vi "VFDSampleSensorLoop.vi"   [LabVIEW 2018]
uses:
  VFDSampleSensorLoopData.ctl
  VFDSampleSensorLoopStates.ctl
  VFDSample.ctl
  VFDErrorSample.ctl
  VFDErrorCodes.ctl
  <vilib>/Platform/TimedLoop/XDataNode/timing_clust.ctl
  <vilib>/Platform/TimedLoop/XDataNode/nitl_modes.ctl
  <vilib>/Platform/TimedLoop/XDataNode/wakeup.ctl
  <vilib>/rvi/Emulation/niFpgaSctlEmulationGetInTimedLoop.vi
  <vilib>/rvi/Emulation/niFpgaEmulationReportErrorSimple.vi
  <vilib>/rvi/Emulation/niFpgaGetClockAttributes.vi
  <vilib>/rvi/Emulation/niFpgaCriticalErrorInLSC.vi
  <vilib>/rvi/Emulation/niFpgaEmulationIsFPGAContextNoSignature.vi
  <vilib>/rvi/errors/niFpgaSetErrorForExecOnDevCompSimple.vi
  <vilib>/rvi/eio/common/nirviEmuReportErrorAndStop.vi
  <vilib>/rvi/DataTransferAndStorage/Container/Common/niFpgaContainerGetUniqueNameForEmu.vi
  <vilib>/rvi/FIFO/Fifo_Resource/nirvififoEmulationSetSize.vi
  <vilib>/rvi/FIFO/Fifo_Resource/nirviFifoEmulationQueueMgr.vi
  <instcachedir>/0/nirviFifoEmulationQueueMgr_E5CAEC123FF24DC58D834DCA3CDAA9B5.lvgen/nirviFifoEmulationQueueMgr_E5CAEC123FF24DC58D834DCA3CDAA9B5_002.vi
  <vilib>/Utility/error.llb/Clear Errors.vi
  <vilib>/rvi/FIFO/Fifo_Resource/nirvififoEmulationCreateLock.vi
  <vilib>/rvi/Emulation/niFpgaProcessEmulError.vi
  <vilib>/rvi/FIFO/Fifo_Resource/nirvififoEmulationObtainLock.vi
  <vilib>/rvi/FIFO/Fifo_Resource/nirvififoEmulationReleaseLock.vi
  <vilib>/rvi/occurrence/nirviWaitOnOccurrenceBase.vi
  <vilib>/rvi/errors/nirviReportUnexpectedCaseInternalError.vi
  <vilib>/rvi/errors/nirviReportUnexpectedCaseInternalError (U32).vi
  <vilib>/rvi/FIFO/Fifo_Resource/nirvififoEmulationDetermineInputValidOut.vi
  <instcachedir>/0/nirviFifoEmulationQueueMgr_E5CAEC123FF24DC58D834DCA3CDAA9B5.lvgen/nirviFifoEmulationQueueMgr_E5CAEC123FF24DC58D834DCA3CDAA9B5_001.vi
  <instcachedir>/0/nirviFifoEmulationQueueMgr_E5CAEC123FF24DC58D834DCA3CDAA9B5.lvgen/nirviFifoEmulationQueueMgr_E5CAEC123FF24DC58D834DCA3CDAA9B5_004.vi
  <vilib>/rvi/Memory/Memory_Emulation/niFpgaMemoryEmulationCacheClearOnFirstRun.vi
  <vilib>/rvi/Memory/Memory_Emulation/nirvimemoryEmulationManagerCache_MakeExclusive.vi
  <vilib>/rvi/Memory/Memory_Emulation/niFpgaMemoryEmulationValidateCache.vi
  <vilib>/rvi/Memory/Memory_Emulation/nirvimemoryEmulationManagerCache_InsertValue.vi
  <vilib>/rvi/Memory/Memory_Emulation/nirvimemoryEmulationManagerCache_ReleaseExclusive.vi
  <vilib>/rvi/Memory/Memory_Emulation/nirvimemoryEmulationManagerCache_GetValue.vi
  <vilib>/rvi/Memory/Memory_Emulation/nirvimemoryEmulationManagerCache_SetValue.vi
  <instcachedir>/0/nirviFifoEmulationQueueMgr_E5CAEC123FF24DC58D834DCA3CDAA9B5.lvgen/nirviFifoEmulationQueueMgr_E5CAEC123FF24DC58D834DCA3CDAA9B5_029.vi
  <instcachedir>/0/nirviFifoEmulationQueueMgr_E5CAEC123FF24DC58D834DCA3CDAA9B5.lvgen/nirviFifoEmulationQueueMgr_E5CAEC123FF24DC58D834DCA3CDAA9B5_015.vi
  <vilib>/Platform/TimedLoop/XDataNode/XDataNode.xnode
  <vilib>/rvi/DataTransferAndStorage/Container/XNode/niFpgaContainer.xnode
  <vilib>/rvi/FIFO/Fifo_Resource/nirvififoEmulationRead.vi
  <vilib>/rvi/FIFO/Fifo_Resource/nirvififoEmulationWrite.vi
  <vilib>/rvi/DataTransferAndStorage/Register/Emulation/niFpgaRegisterEmulation.vi
  <vilib>/Platform/TimedLoop/XDataNode/XDNodeRunTimeDep.lvlib
types:
  T1 = typedef "VFDSampleSensorLoopData.ctl" = cluster{"State":T2, "StateAfterRead":T2, "Timestamp":u64, "Timeout":i32, "U16":u16, "CRC":u16, "Exception":u8, "Sample":T3, "ErrorSample":T4}
  T2 = typedef "VFDSampleSensorLoopStates.ctl" = enum16{"WaitForTrigger", "ClearRxFIFO", "WaitForClearComplete", "WriteAddress", "WriteFunction", "WriteStartAddress1", "WriteStartAddress0", "WriteAddressCount1", "WriteAddressCount0", "WriteCRC1", "WriteCRC0", "ReadAddress", "ReadFunction", "ReadByteCount", "StartVelocityBits", "EndVelocityBits", "StartDriveErrorBits", "EndDriveErrorBits", "StartFrequencyCommand", "EndFrequencyCommand", "StartOutputFrequency", "EndOutputFrequency", "StartOutputCurrent", "EndOutputCurrent", "StartDCBusVoltage", "EndDCBusVoltage", "StartOutputVoltage", "EndOutputVoltage", "ReadDataByte1", "ReadDataByte0", "Reserved1", "Reserved2", "ReadCRCByte0", "ReadCRCByte1", "CalculateCRC", "ValidateCRC", "PrepareSample", "MoveSample", "ReadExceptionCode", "ReadExceptionCRCByte0", "ReadExceptionCRCByte1", "CalculateExceptionCRC", "ValidateExceptionCRC", "ParseExceptionCode", "ResponseAddressError", "ResponseFunctionCodeError", "ResponseByteCountError", "ResponseCRCError", "ResponseUnknownError", "ResponseTimeoutError", "SensorReportsIllegalFunction", "SensorReportsIllegalDataAddress", "PrepareErrorCode", "MoveErrorCode", "WriteDemandAddress", "WriteDemandFunction", "WriteDemandStartAddress1", "WriteDemandStartAddress0", "WriteDemandData1", "WriteDemandData0", "CalculateDemandCRC", "WaitForDemandCRC", "WriteDemandCRC1", "WriteDemandCRC0", "ReadDemandAddress", "ReadDemandFunction", "ReadDemandStartAddress1", "ReadDemandStartAddress0", "ReadDemandData1", "ReadDemandData0", "ReadDemandCRC0", "ReadDemandCRC1", "CalculateDemandResponseCRC", "ValidateDemandResponseCRC"}
  T3 = typedef "VFDSample.ctl" = cluster{"Timestamp":u64, "TxBytes":u64, "RxBytes":u64, "TxFrames":u64, "RxFrames":u64, "VelocityBits":u16, "DriveErrorBits":u16, "FrequencyCommand":u16, "OutputFrequency":u16, "OutputCurrent":u16, "DCBusVoltage":u16, "OutputVoltage":u16}
  T4 = typedef "VFDErrorSample.ctl" = cluster{"Timestamp":u64, "TxBytes":u64, "RxBytes":u64, "TxFrames":u64, "RxFrames":u64, "ErrorCode":T5}
  T5 = typedef "VFDErrorCodes.ctl" = enum8{"None", "ResponseAddressError", "ResponseFunctionCodeError", "ResponseByteCountError", "ResponseCRCError", "ResponseUnknownError", "ResponseTimeoutError", "SensorReportsIllegalFunction", "SensorReportsIllegalDataAddress"}
  T6 = typedef "XDNodeRunTimeDep.lvlib/timing_clust.ctl" = cluster{"Expected End [f-1]":u64, "Actual End [f-1]":u64, "Finished Late? [f-1]":bool, "Expected End [i-1]":u64, "Actual End [i-1]":u64, "Finished Late? [i-1]":bool, "Expected Start [i]":u64, "Actual Start [i]":u64, "Expected Start [f]":u64, "Actual Start [f]":u64, "Source Name":string, "Structure Name":string, "Period":i64, "Deadline":i64, "Offset":i64, "Start":i64, "Priority":i32, "Timeout":i32, "Mode":T7, "Wakeup Reason":T8, "Error":errorcluster, "Source Type":string, "Secondary Source Type":string, "Global End Time":u64, "Global Start Time":u64, "Frame Duration":u64, "Iteration Duration":u64, "Assigned CPU":i32, "I/O Scan Engine Mode":u32}
  T7 = typedef "XDNodeRunTimeDep.lvlib/nitl_modes.ctl" = enum32{"No Change", "Process missed periods, maintain original phase", "Discard missed periods, maintain original phase", "Process missed periods, ignore original phase", "Discard missed periods, ignore original phase"}
  T8 = typedef "XDNodeRunTimeDep.lvlib/wakeup.ctl" = enum32{"Normal", "Aborted", "Asynchronous wakeup", "Timing source error", "Timed loop error", "Timeout"}
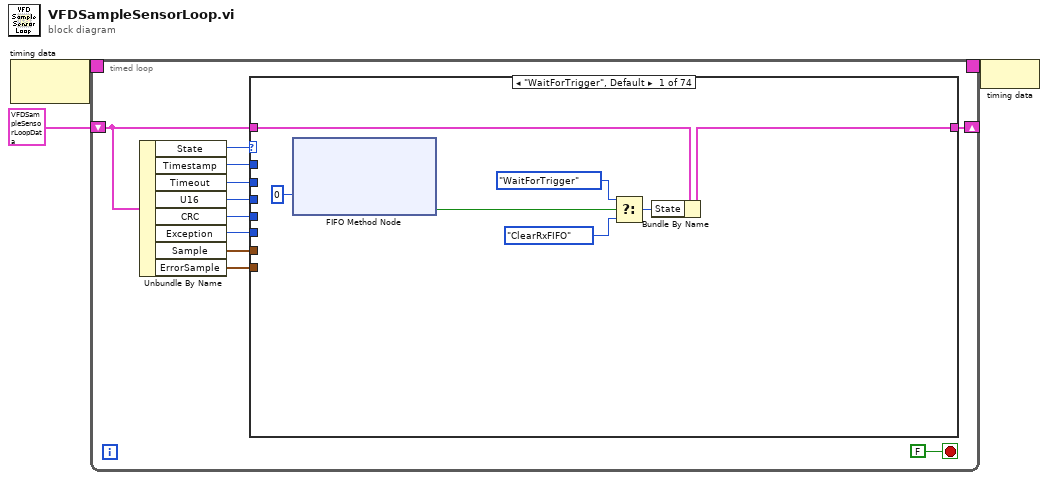
[diagram p0: block diagram]
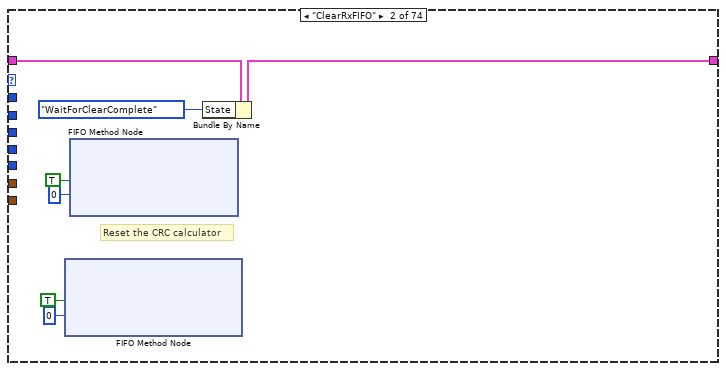
[diagram p2: hidden frame]
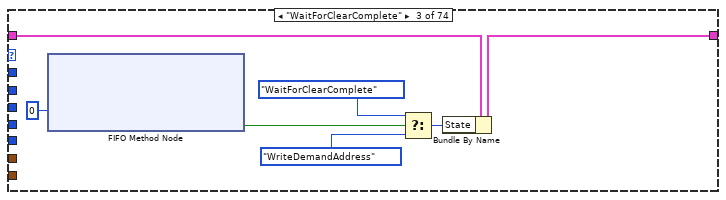
[diagram p3: hidden frame]
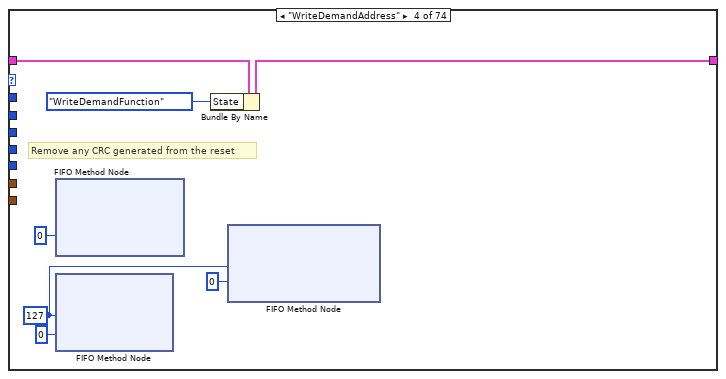
[diagram p4: hidden frame]
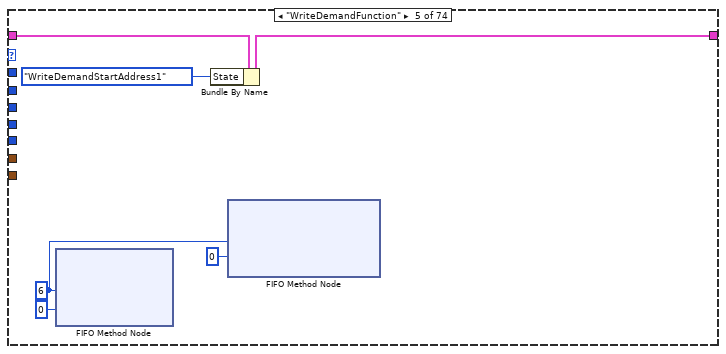
[diagram p5: hidden frame]
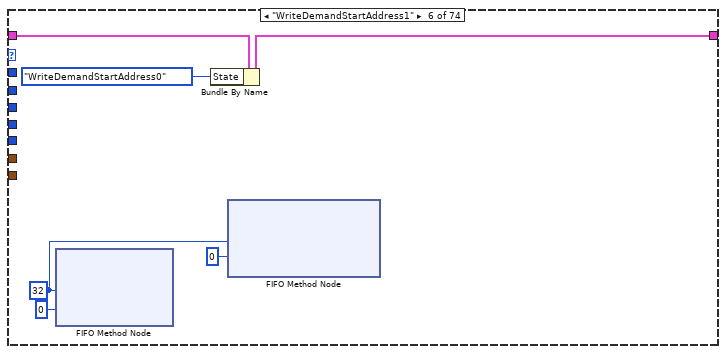
[diagram p6: hidden frame]
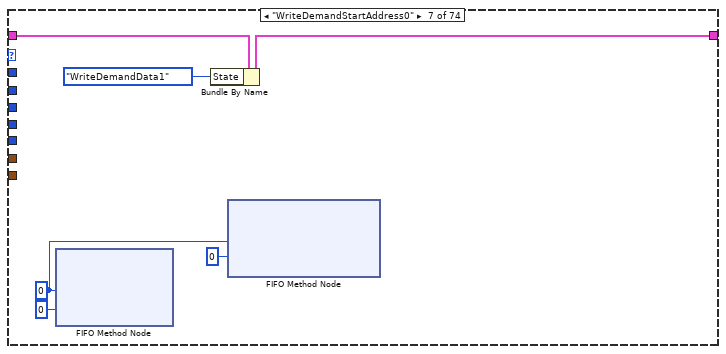
[diagram p7: hidden frame]
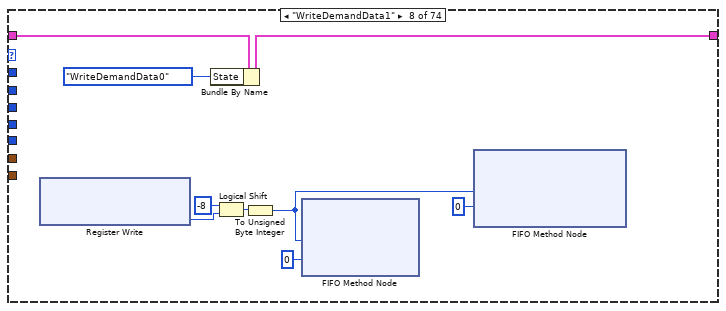
[diagram p8: hidden frame]
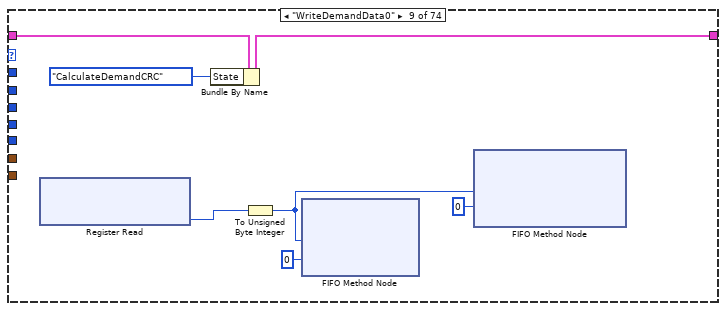
[diagram p9: hidden frame]
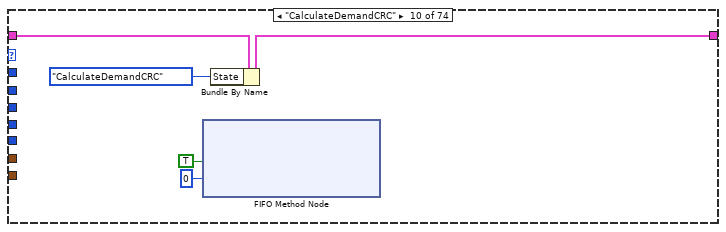
[diagram p10: hidden frame]
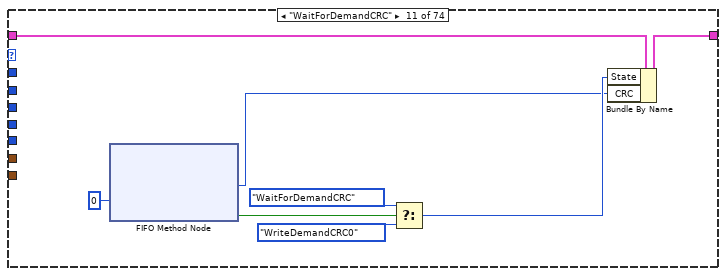
[diagram p11: hidden frame]
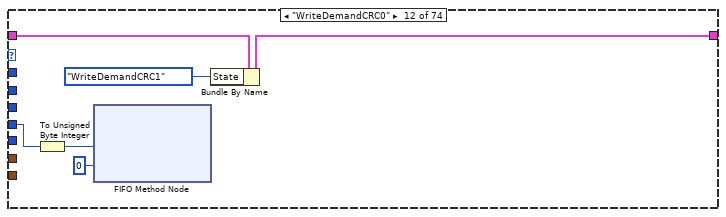
[diagram p12: hidden frame]
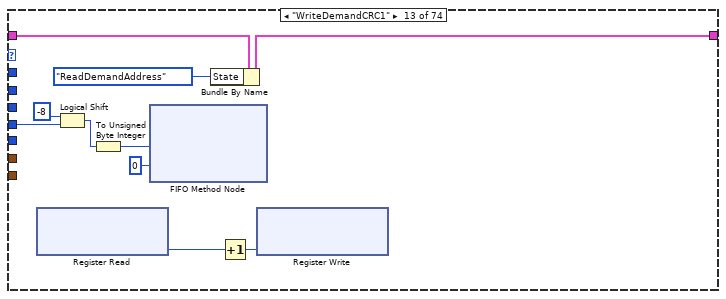
[diagram p13: hidden frame]
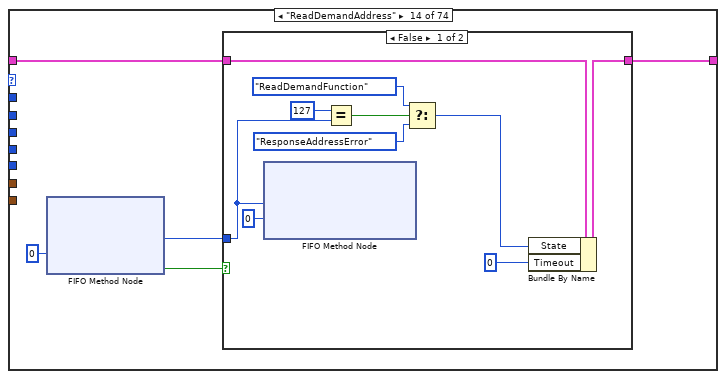
[diagram p14: hidden frame]
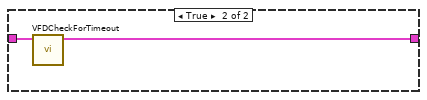
[diagram p15: hidden frame]
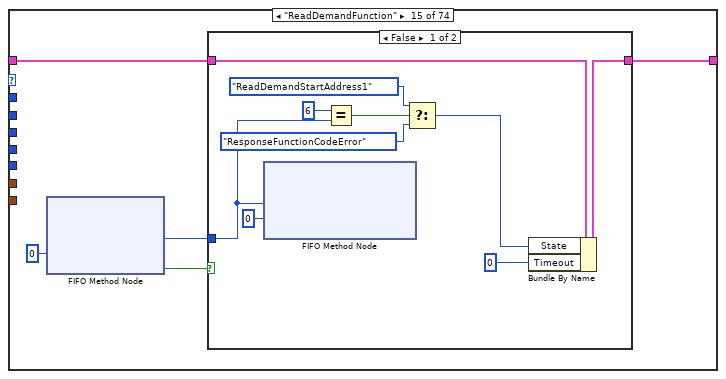
[diagram p16: hidden frame]
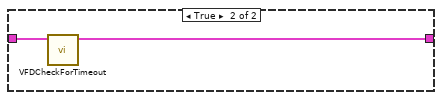
[diagram p17: hidden frame]
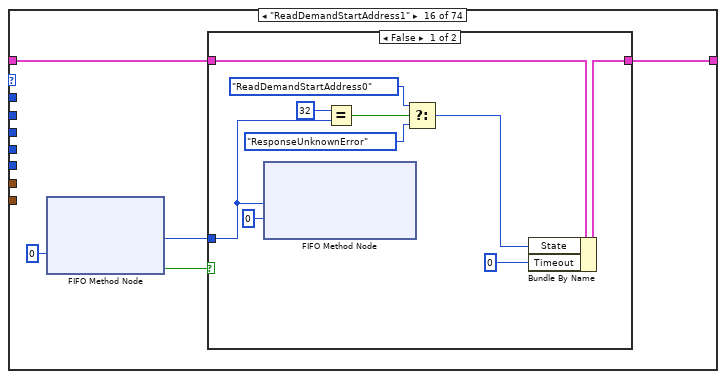
[diagram p18: hidden frame]
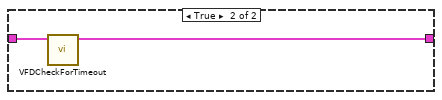
[diagram p19: hidden frame]
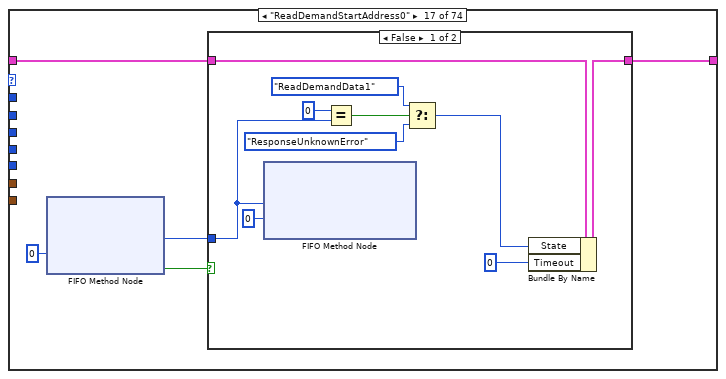
[diagram p20: hidden frame]
diagram:
  n1 = node-c288() -> (w3:T6)  [unwired: 1 in]
  n2 = timed-loop {
    timing: w3 -> [_]
    timing-out: [_] -> w2
    shift-right: [w13] -> _
    shift-left: T1 {"State"=enum."WaitForTrigger", "StateAfterRead"=enum."ClearRxFIFO", "Timestamp"=0, "Timeout"=0, "U16"=0, "CRC"=0, "Exception"=0, "Sample"={"Timestamp"=0, "TxBytes"=0, "RxBytes"=0, "TxFrames"=0, "RxFrames"=0, "VelocityBits"=0, "DriveErrorBits"=0, "FrequencyCommand"=0, "OutputFrequency"=0, "OutputCurrent"=0, "DCBusVoltage"=0, "OutputVoltage"=0}, "ErrorSample"={"Timestamp"=0, "TxBytes"=0, "RxBytes"=0, "TxFrames"=0, "RxFrames"=0, "ErrorCode"=enum."None"}} ("InclinometerData") -> [w14]
    stop <- FALSE stop-if-true
    n3 = Unbundle By Name(w14) -> ("State"=w12:T2, "Timestamp"=w7:u64, "Timeout"=w11:i32, "U16"=w10:u16, "CRC"=w9:u16, "Exception"=w6:u8, "Sample"=w5:T3, "ErrorSample"=w4:T4)
    n4 = case shown="\"WaitForTrigger\", Default" w12 {
      tunnel: w14 -> [w20 w27 w34 w41 w47 w53 w59 w68 w75 w80 w88 w94 w104 w106 w123 w140 w157 w174 w194 w212 w227 w247 w250 w271 w276 w281 w286 w291 w296 w301 w309 w313 w330 w351 w372 w376 w381 w385 w390 w394 w399 w403 w408 w412 w417 w421 w426 w430 w432 w455 w474 w477 w482 w502 w522 w527 w547 w552 w556 w577 w597 w617 w622 w642 w646 w650 w654 w658 w662 w666 w670 w674 w682 w687]
      tunnel: [w21 w28 w35 w42 w48 w54 w60 w69 w76 w81 w89 w95 w105 w107 w124 w141 w158 w175 w195 w213 w228 w245 w251 w272 w277 w282 w287 w292 w297 w302 w310 w314 w331 w352 w371 w375 w380 w384 w389 w393 w398 w402 w407 w411 w416 w420 w425 w429 w433 w456 w475 w478 w483 w503 w523 w528 w548 w553 w557 w578 w598 w618 w623 w643 w647 w651 w655 w659 w663 w667 w671 w675 w683 w688] -> w13
      tunnel: w11 -> [_ _ _ _ _ _ _ _ _ _ _ _ _ _ _ _ _ _ _ _ _ _ _ _ _ _ _ _ _ _ _ _ _ _ _ _ _ _ _ _ _ _ _ _ _ _ _ _ _ _ _ _ _ _ _ _ _ _ _ _ _ _ _ _ _ _ _ _ _ _ _ _ _ _]
      tunnel: w10 -> [_ _ _ _ _ _ _ _ _ _ _ _ _ _ _ _ _ _ _ _ _ _ _ _ _ _ _ _ _ _ _ _ _ _ _ w373 _ w382 _ w391 _ w400 _ w409 _ w418 _ w427 w431 w454 _ _ _ _ _ _ _ _ _ _ _ _ _ _ _ _ _ _ _ _ _ _ _ _]
      tunnel: w9 -> [_ _ _ _ _ _ _ _ _ _ _ w90 w100 _ _ _ _ _ _ _ w226 _ w249 _ _ _ _ _ _ _ _ _ _ _ _ _ _ _ _ _ _ _ _ _ _ _ _ _ _ _ _ _ w481 w501 _ w526 _ _ _ w576 w596 _ w621 _ _ _ _ _ _ _ _ _ _ _]
      tunnel: w7 -> [_ _ _ _ _ _ _ _ _ _ _ _ _ _ _ _ _ _ _ _ _ _ _ _ _ _ _ _ _ _ _ _ _ _ _ _ _ _ _ _ _ _ _ _ _ _ _ _ _ _ _ _ _ _ _ _ w546 _ _ _ _ _ _ _ _ _ _ _ _ _ _ _ w681 _]
      tunnel: w6 -> [_ _ _ _ _ _ _ _ _ _ _ _ _ _ _ _ _ _ _ _ _ _ _ _ _ _ _ _ _ _ _ _ _ _ _ _ _ _ _ _ _ _ _ _ _ _ _ _ _ _ _ _ _ _ _ _ _ _ _ _ _ _ _ w637 _ _ _ _ _ _ _ _ _ _]
      tunnel: w5 -> [_ _ _ _ _ _ _ _ _ _ _ _ _ _ _ _ _ _ _ _ _ _ _ _ _ _ _ _ _ _ _ _ _ _ _ _ _ _ _ _ _ _ _ _ _ _ _ _ _ _ _ _ _ _ _ _ _ w549 _ _ _ _ _ _ _ _ _ _ _ _ _ _ _ _]
      tunnel: w4 -> [_ _ _ _ _ _ _ _ _ _ _ _ _ _ _ _ _ _ _ _ _ _ _ _ _ _ _ _ _ _ _ _ _ _ _ _ _ _ _ _ _ _ _ _ _ _ _ _ _ _ _ _ _ _ _ _ _ _ _ _ _ _ _ _ _ _ _ _ _ _ _ _ _ w685]
      frame "WaitForTrigger", Default {
        n5 = xnode ("FIFO Method Node")("Timeout"=0) -> ("Timed Out?"=w15:bool)  [unwired: 1 in, 2 out]
        n6 = Select(t=VFDSampleSensorLoopStates."WaitForTrigger" ("InclinometerState"), s=w15, f=VFDSampleSensorLoopStates."ClearRxFIFO" ("InclinometerState")) -> (s? t:f=w17:T2)
        n7 = Bundle By Name(cluster=w20, "State"=w17) -> (w21:T1)
      }
      frame "ClearRxFIFO" {
        # "Reset the CRC calculator"
        n8 = xnode ("FIFO Method Node")("Element"=TRUE, "Timeout"=0) -> ()  [unwired: 1 in, 2 out]
        n9 = xnode ("FIFO Method Node")("Element"=TRUE, "Timeout"=0) -> ()  [unwired: 1 in, 2 out]
        n10 = Bundle By Name(cluster=w27, "State"=VFDSampleSensorLoopStates."WaitForClearComplete" ("InclinometerState")) -> (w28:T1)
      }
      frame "WaitForClearComplete" {
        n11 = xnode ("FIFO Method Node")("Timeout"=0) -> ("Timed Out?"=w29:bool)  [unwired: 1 in, 2 out]
        n12 = Select(t=VFDSampleSensorLoopStates."WaitForClearComplete", s=w29, f=VFDSampleSensorLoopStates."WriteDemandAddress" ("InclinometerState")) -> (s? t:f=w31:T2)
        n13 = Bundle By Name(cluster=w34, "State"=w31) -> (w35:T1)
      }
      frame "WriteDemandAddress" {
        w37 = u8 127 ("Element")
        # "Remove any CRC generated from the reset"
        n14 = xnode ("FIFO Method Node")("Timeout"=0) -> ()  [unwired: 1 in, 3 out]
        n15 = xnode ("FIFO Method Node")("Element"=w37, "Timeout"=0) -> ()  [unwired: 1 in, 2 out]
        n16 = Bundle By Name(cluster=w41, "State"=VFDSampleSensorLoopStates."WriteDemandFunction" ("InclinometerState")) -> (w42:T1)
        n17 = xnode ("FIFO Method Node")("Element"=w37, "Timeout"=0) -> ()  [unwired: 1 in, 2 out]
      }
      frame "WriteDemandFunction" {
        w44 = u8 6 ("Element")
        n18 = xnode ("FIFO Method Node")("Element"=w44, "Timeout"=0) -> ()  [unwired: 1 in, 2 out]
        n19 = Bundle By Name(cluster=w47, "State"=VFDSampleSensorLoopStates."WriteDemandStartAddress1" ("InclinometerState")) -> (w48:T1)
        n20 = xnode ("FIFO Method Node")("Element"=w44, "Timeout"=0) -> ()  [unwired: 1 in, 2 out]
      }
      frame "WriteDemandStartAddress1" {
        w50 = u8 32 ("Element")
        n21 = xnode ("FIFO Method Node")("Element"=w50, "Timeout"=0) -> ()  [unwired: 1 in, 2 out]
        n22 = Bundle By Name(cluster=w53, "State"=VFDSampleSensorLoopStates."WriteDemandStartAddress0" ("InclinometerState")) -> (w54:T1)
        n23 = xnode ("FIFO Method Node")("Element"=w50, "Timeout"=0) -> ()  [unwired: 1 in, 2 out]
      }
      frame "WriteDemandStartAddress0" {
        w56 = u8 0 ("Element")
        n24 = xnode ("FIFO Method Node")("Element"=w56, "Timeout"=0) -> ()  [unwired: 1 in, 2 out]
        n25 = Bundle By Name(cluster=w59, "State"=VFDSampleSensorLoopStates."WriteDemandData1" ("InclinometerState")) -> (w60:T1)
        n26 = xnode ("FIFO Method Node")("Element"=w56, "Timeout"=0) -> ()  [unwired: 1 in, 2 out]
      }
      frame "WriteDemandData1" {
        n27 = xnode "Register Write"() -> ("Data"=w64:u16)  [unwired: 1 in, 1 out]
        n28 = Bundle By Name(cluster=w68, "State"=VFDSampleSensorLoopStates."WriteDemandData0" ("InclinometerState")) -> (w69:T1)
        n29 = Logical Shift(y=i16 -8, x=w64) -> (x << y=w62:u16)
        n30 = To Unsigned Byte Integer(number=w62) -> (unsigned 8bit integer=w61:u8)
        n31 = xnode ("FIFO Method Node")("Element"=w61, "Timeout"=0) -> ()  [unwired: 1 in, 2 out]
        n32 = xnode ("FIFO Method Node")("Element"=w61, "Timeout"=0) -> ()  [unwired: 1 in, 2 out]
      }
      frame "WriteDemandData0" {
        n33 = xnode "Register Read"() -> ("Data"=w70:u16)  [unwired: 1 in, 1 out]
        n34 = Bundle By Name(cluster=w75, "State"=VFDSampleSensorLoopStates."CalculateDemandCRC" ("InclinometerState")) -> (w76:T1)
        n35 = To Unsigned Byte Integer(number=w70) -> (unsigned 8bit integer=w71:u8)
        n36 = xnode ("FIFO Method Node")("Element"=w71, "Timeout"=0) -> ()  [unwired: 1 in, 2 out]
        n37 = xnode ("FIFO Method Node")("Element"=w71, "Timeout"=0) -> ()  [unwired: 1 in, 2 out]
      }
      frame "CalculateDemandCRC" {
        n38 = xnode ("FIFO Method Node")("Element"=TRUE, "Timeout"=0) -> ()  [unwired: 1 in, 2 out]
        n39 = Bundle By Name(cluster=w80, "State"=VFDSampleSensorLoopStates."CalculateDemandCRC" ("InclinometerState")) -> (w81:T1)
      }
      frame "WaitForDemandCRC" {
        n40 = xnode ("FIFO Method Node")("Timeout"=0) -> ("Element"=w82:u16, "Timed Out?"=w87:bool)  [unwired: 1 in, 1 out]
        n41 = Select(t=VFDSampleSensorLoopStates."WaitForDemandCRC", s=w87, f=VFDSampleSensorLoopStates."WriteDemandCRC0" ("InclinometerState")) -> (s? t:f=w83:T2)
        n42 = Bundle By Name(cluster=w88, "State"=w83, "CRC"=w82) -> (w89:T1)
      }
      frame "WriteDemandCRC0" {
        n43 = To Unsigned Byte Integer(number=w90) -> (unsigned 8bit integer=w91:u8)
        n44 = xnode ("FIFO Method Node")("Element"=w91, "Timeout"=0) -> ()  [unwired: 1 in, 2 out]
        n45 = Bundle By Name(cluster=w94, "State"=VFDSampleSensorLoopStates."WriteDemandCRC1" ("InclinometerState")) -> (w95:T1)
      }
      frame "WriteDemandCRC1" {
        n46 = xnode ("Register Read")() -> ("Data"=w97:u64)  [unwired: 1 in, 1 out]
        n47 = Logical Shift(y=i16 -8, x=w100) -> (x << y=w98:u16)
        n48 = To Unsigned Byte Integer(number=w98) -> (unsigned 8bit integer=w101:u8)
        n49 = xnode ("FIFO Method Node")("Element"=w101, "Timeout"=0) -> ()  [unwired: 1 in, 2 out]
        n50 = Bundle By Name(cluster=w104, "State"=VFDSampleSensorLoopStates."ReadDemandAddress" ("InclinometerState")) -> (w105:T1)
        n51 = Increment(x=w97) -> (x+1=w96:u64)
        n52 = xnode ("Register Write")("Data"=w96) -> ()  [unwired: 1 in, 1 out]
      }
      frame "ReadDemandAddress" {
        n53 = xnode ("FIFO Method Node")("Timeout"=0) -> ("Element"=w108:u8, "Timed Out?"=w109:bool)  [unwired: 1 in, 1 out]
        n54 = case shown="False" w109 {
          tunnel: w108 -> [w117 _]
          tunnel: [w119 w121] -> w107
          tunnel: w106 -> [w120 w122]
          frame False {
            n55 = xnode ("FIFO Method Node")("Element"=w117, "Timeout"=0) -> ()  [unwired: 1 in, 2 out]
            n56 = Equal?(x=u8 127, y=w117) -> (x = y?=w115:bool)
            n57 = Select(t=VFDSampleSensorLoopStates."ReadDemandFunction" ("InclinometerState"), s=w115, f=VFDSampleSensorLoopStates."ResponseAddressError" ("InclinometerState")) -> (s? t:f=w112:T2)
            n58 = Bundle By Name(cluster=w120, "State"=w112, "Timeout"=0) -> (w119:T1)
          }
          frame True {
            n59 = call "VFDCheckForTimeout.vi"("VFDSampleSensorLoopData in"=w122) -> ("VFDSampleSensorLoopData out"=w121:T1)  [unwired: 10 in]
          }
        }
      }
      frame "ReadDemandFunction" {
        n60 = xnode ("FIFO Method Node")("Timeout"=0) -> ("Element"=w125:u8, "Timed Out?"=w126:bool)  [unwired: 1 in, 1 out]
        n61 = case shown="False" w126 {
          tunnel: w125 -> [w134 _]
          tunnel: [w136 w138] -> w124
          tunnel: w123 -> [w137 w139]
          frame False {
            n62 = xnode ("FIFO Method Node")("Element"=w134, "Timeout"=0) -> ()  [unwired: 1 in, 2 out]
            n63 = Equal?(x=u8 6, y=w134) -> (x = y?=w132:bool)
            n64 = Select(t=VFDSampleSensorLoopStates."ReadDemandStartAddress1" ("InclinometerState"), s=w132, f=VFDSampleSensorLoopStates."ResponseFunctionCodeError" ("InclinometerState")) -> (s? t:f=w129:T2)
            n65 = Bundle By Name(cluster=w137, "State"=w129, "Timeout"=0) -> (w136:T1)
          }
          frame True {
            n66 = call "VFDCheckForTimeout.vi"("VFDSampleSensorLoopData in"=w139) -> ("VFDSampleSensorLoopData out"=w138:T1)  [unwired: 10 in]
          }
        }
      }
      frame "ReadDemandStartAddress1" {
        n67 = xnode ("FIFO Method Node")("Timeout"=0) -> ("Element"=w142:u8, "Timed Out?"=w143:bool)  [unwired: 1 in, 1 out]
        n68 = case shown="False" w143 {
          tunnel: w142 -> [w151 _]
          tunnel: [w153 w155] -> w141
          tunnel: w140 -> [w154 w156]
          frame False {
            n69 = xnode ("FIFO Method Node")("Element"=w151, "Timeout"=0) -> ()  [unwired: 1 in, 2 out]
            n70 = Equal?(x=u8 32, y=w151) -> (x = y?=w149:bool)
            n71 = Select(t=VFDSampleSensorLoopStates."ReadDemandStartAddress0" ("InclinometerState"), s=w149, f=VFDSampleSensorLoopStates."ResponseUnknownError" ("InclinometerState")) -> (s? t:f=w146:T2)
            n72 = Bundle By Name(cluster=w154, "State"=w146, "Timeout"=0) -> (w153:T1)
          }
          frame True {
            n73 = call "VFDCheckForTimeout.vi"("VFDSampleSensorLoopData in"=w156) -> ("VFDSampleSensorLoopData out"=w155:T1)  [unwired: 10 in]
          }
        }
      }
      frame "ReadDemandStartAddress0" {
        n74 = xnode ("FIFO Method Node")("Timeout"=0) -> ("Element"=w159:u8, "Timed Out?"=w160:bool)  [unwired: 1 in, 1 out]
        n75 = case shown="False" w160 {
          tunnel: w159 -> [w168 _]
          tunnel: [w170 w172] -> w158
          tunnel: w157 -> [w171 w173]
          frame False {
            n76 = xnode ("FIFO Method Node")("Element"=w168, "Timeout"=0) -> ()  [unwired: 1 in, 2 out]
            n77 = Equal?(x=u8 0, y=w168) -> (x = y?=w166:bool)
            n78 = Select(t=VFDSampleSensorLoopStates."ReadDemandData1" ("InclinometerState"), s=w166, f=VFDSampleSensorLoopStates."ResponseUnknownError" ("InclinometerState")) -> (s? t:f=w163:T2)
            n79 = Bundle By Name(cluster=w171, "State"=w163, "Timeout"=0) -> (w170:T1)
          }
          frame True {
            n80 = call "VFDCheckForTimeout.vi"("VFDSampleSensorLoopData in"=w173) -> ("VFDSampleSensorLoopData out"=w172:T1)  [unwired: 10 in]
          }
        }
      }
      frame "ReadDemandData1" {
        n81 = xnode ("FIFO Method Node")("Timeout"=0) -> ("Element"=w176:u8, "Timed Out?"=w177:bool)  [unwired: 1 in, 1 out]
        n82 = case shown="False" w177 {
          tunnel: w176 -> [w188 _]
          tunnel: [w190 w192] -> w175
          tunnel: w174 -> [w191 w193]
          frame False {
            n83 = xnode "Register Write"() -> ("Data"=w182:u16)  [unwired: 1 in, 1 out]
            n84 = Logical Shift(y=i16 -8, x=w182) -> (x << y=w180:u16)
            n85 = xnode ("FIFO Method Node")("Element"=w188, "Timeout"=0) -> ()  [unwired: 1 in, 2 out]
            n86 = To Unsigned Byte Integer(number=w180) -> (unsigned 8bit integer=w179:u8)
            n87 = Equal?(x=w179, y=w188) -> (x = y?=w187:bool)
            n88 = Select(t=VFDSampleSensorLoopStates."ReadDemandData0" ("InclinometerState"), s=w187, f=VFDSampleSensorLoopStates."ResponseUnknownError" ("InclinometerState")) -> (s? t:f=w184:T2)
            n89 = Bundle By Name(cluster=w191, "State"=w184, "Timeout"=0) -> (w190:T1)
          }
          frame True {
            n90 = call "VFDCheckForTimeout.vi"("VFDSampleSensorLoopData in"=w193) -> ("VFDSampleSensorLoopData out"=w192:T1)  [unwired: 10 in]
          }
        }
      }
      frame "ReadDemandData0" {
        n91 = xnode ("FIFO Method Node")("Timeout"=0) -> ("Element"=w196:u8, "Timed Out?"=w197:bool)  [unwired: 1 in, 1 out]
        n92 = case shown="False" w197 {
          tunnel: w196 -> [w206 _]
          tunnel: [w208 w210] -> w195
          tunnel: w194 -> [w209 w211]
          frame False {
            n93 = xnode "Register Read"() -> ("Data"=w199:u16)  [unwired: 1 in, 1 out]
            n94 = xnode ("FIFO Method Node")("Element"=w206, "Timeout"=0) -> ()  [unwired: 1 in, 2 out]
            n95 = To Unsigned Byte Integer(number=w199) -> (unsigned 8bit integer=w200:u8)
            n96 = Equal?(x=w200, y=w206) -> (x = y?=w205:bool)
            n97 = Select(t=VFDSampleSensorLoopStates."ReadDemandCRC0" ("InclinometerState"), s=w205, f=VFDSampleSensorLoopStates."ResponseUnknownError" ("InclinometerState")) -> (s? t:f=w202:T2)
            n98 = Bundle By Name(cluster=w209, "State"=w202, "Timeout"=0) -> (w208:T1)
          }
          frame True {
            n99 = call "VFDCheckForTimeout.vi"("VFDSampleSensorLoopData in"=w211) -> ("VFDSampleSensorLoopData out"=w210:T1)  [unwired: 10 in]
          }
        }
      }
      frame "ReadDemandCRC0" {
        n100 = xnode ("FIFO Method Node")("Timeout"=0) -> ("Element"=w214:u8, "Timed Out?"=w215:bool)  [unwired: 1 in, 1 out]
        n101 = case shown="False" w215 {
          tunnel: w214 -> [w217 _]
          tunnel: [w221 w223] -> w213
          tunnel: w212 -> [w222 w224]
          frame False {
            n102 = To Unsigned Word Integer(number=w217) -> (unsigned 16bit integer=w218:u16)
            n103 = Bundle By Name(cluster=w222, "State"=VFDSampleSensorLoopStates."ReadDemandCRC1" ("InclinometerState"), "Timeout"=0, "CRC"=w218) -> (w221:T1)
          }
          frame True {
            n104 = call "VFDCheckForTimeout.vi"("VFDSampleSensorLoopData in"=w224) -> ("VFDSampleSensorLoopData out"=w223:T1)  [unwired: 10 in]
          }
        }
      }
      frame "ReadDemandCRC1" {
        n105 = xnode ("FIFO Method Node")("Timeout"=0) -> ("Element"=w225:u8, "Timed Out?"=w229:bool)  [unwired: 1 in, 1 out]
        n106 = case shown="False" w229 {
          tunnel: [w239 w241] -> w228
          tunnel: w227 -> [w240 w242]
          tunnel: w226 -> [w232 _]
          tunnel: w225 -> [w236 _]
          frame False {
            n107 = To Unsigned Word Integer(number=w236) -> (unsigned 16bit integer=w235:u16)
            n108 = Logical Shift(y=i16 8, x=w235) -> (x << y=w233:u16)
            n109 = Or(x=w232, y=w233) -> (x .or. y?=w231:u16)
            n110 = Bundle By Name(cluster=w240, "State"=VFDSampleSensorLoopStates."CalculateDemandResponseCRC" ("InclinometerState"), "Timeout"=0, "CRC"=w231) -> (w239:T1)
          }
          frame True {
            n111 = call "VFDCheckForTimeout.vi"("VFDSampleSensorLoopData in"=w242) -> ("VFDSampleSensorLoopData out"=w241:T1)  [unwired: 10 in]
          }
        }
      }
      frame "CalculateDemandResponseCRC" {
        n112 = xnode ("FIFO Method Node")("Element"=TRUE, "Timeout"=0) -> ()  [unwired: 1 in, 2 out]
        n113 = Bundle By Name(cluster=w247, "State"=VFDSampleSensorLoopStates."ValidateDemandResponseCRC") -> (w245:T1)
      }
      frame "ValidateDemandResponseCRC" {
        n114 = xnode ("FIFO Method Node")("Timeout"=0) -> ("Element"=w248:u16, "Timed Out?"=w252:bool)  [unwired: 1 in, 1 out]
        n115 = case shown="False" w252 {
          tunnel: [w263 w265] -> w251
          tunnel: w250 -> [w264 w266]
          tunnel: w249 -> [w261 _]
          tunnel: w248 -> [w260 _]
          frame False {
            n116 = xnode ("Register Read")() -> ("Data"=w255:u64)  [unwired: 1 in, 1 out]
            n117 = Equal?(x=w261, y=w260) -> (x = y?=w259:bool)
            n118 = Increment(x=w255) -> (x+1=w254:u64)
            n119 = Select(t=VFDSampleSensorLoopStates."ReadAddress" ("InclinometerState"), s=w259, f=VFDSampleSensorLoopStates."ResponseCRCError") -> (s? t:f=w256:T2)
            n120 = xnode ("Register Write")("Data"=w254) -> ()  [unwired: 1 in, 1 out]
            n121 = Bundle By Name(cluster=w264, "State"=w256, "Timeout"=0) -> (w263:T1)
          }
          frame True {
            n122 = call "VFDCheckForTimeout.vi"("VFDSampleSensorLoopData in"=w266) -> ("VFDSampleSensorLoopData out"=w265:T1)  [unwired: 10 in]
          }
        }
      }
      frame "WriteAddress" {
        # "Remove any CRC generated from the reset"
        n123 = xnode ("FIFO Method Node")("Timeout"=0) -> ()  [unwired: 1 in, 3 out]
        n124 = xnode ("FIFO Method Node")("Element"=u8 127, "Timeout"=0) -> ()  [unwired: 1 in, 2 out]
        n125 = Bundle By Name(cluster=w271, "State"=VFDSampleSensorLoopStates."WriteFunction" ("InclinometerState")) -> (w272:T1)
      }
      frame "WriteFunction" {
        n126 = xnode ("FIFO Method Node")("Element"=u8 3, "Timeout"=0) -> ()  [unwired: 1 in, 2 out]
        n127 = Bundle By Name(cluster=w276, "State"=VFDSampleSensorLoopStates."WriteStartAddress1" ("InclinometerState")) -> (w277:T1)
      }
      frame "WriteStartAddress1" {
        n128 = xnode ("FIFO Method Node")("Element"=u8 33, "Timeout"=0) -> ()  [unwired: 1 in, 2 out]
        n129 = Bundle By Name(cluster=w281, "State"=VFDSampleSensorLoopStates."WriteStartAddress0" ("InclinometerState")) -> (w282:T1)
      }
      frame "WriteStartAddress0" {
        n130 = xnode ("FIFO Method Node")("Element"=u8 0, "Timeout"=0) -> ()  [unwired: 1 in, 2 out]
        n131 = Bundle By Name(cluster=w286, "State"=VFDSampleSensorLoopStates."WriteAddressCount1" ("InclinometerState")) -> (w287:T1)
      }
      frame "WriteAddressCount1" {
        n132 = xnode ("FIFO Method Node")("Element"=u8 0, "Timeout"=0) -> ()  [unwired: 1 in, 2 out]
        n133 = Bundle By Name(cluster=w291, "State"=VFDSampleSensorLoopStates."WriteAddressCount0" ("InclinometerState")) -> (w292:T1)
      }
      frame "WriteAddressCount0" {
        n134 = xnode ("FIFO Method Node")("Element"=u8 7, "Timeout"=0) -> ()  [unwired: 1 in, 2 out]
        n135 = Bundle By Name(cluster=w296, "State"=VFDSampleSensorLoopStates."WriteCRC1" ("InclinometerState")) -> (w297:T1)
      }
      frame "WriteCRC1" {
        n136 = xnode ("FIFO Method Node")("Element"=u8 4, "Timeout"=0) -> ()  [unwired: 1 in, 2 out]
        n137 = Bundle By Name(cluster=w301, "State"=VFDSampleSensorLoopStates."WriteCRC0" ("InclinometerState")) -> (w302:T1)
      }
      frame "WriteCRC0" {
        n138 = xnode ("Register Read")() -> ("Data"=w304:u64)  [unwired: 1 in, 1 out]
        n139 = xnode ("FIFO Method Node")("Element"=u8 42, "Timeout"=0) -> ()  [unwired: 1 in, 2 out]
        n140 = Bundle By Name(cluster=w309, "State"=VFDSampleSensorLoopStates."ReadAddress" ("InclinometerState"), "Timeout"=0) -> (w310:T1)
        n141 = Increment(x=w304) -> (x+1=w303:u64)
        n142 = xnode ("Register Write")("Data"=w303) -> ()  [unwired: 1 in, 1 out]
      }
      frame "ReadAddress" {
        n143 = xnode "Register Write"() -> ("Data"=w311:u64)  [unwired: 1 in, 1 out]
        n144 = xnode ("FIFO Method Node")("Timeout"=0) -> ("Element"=w315:u8, "Timed Out?"=w316:bool)  [unwired: 1 in, 1 out]
        n145 = Bundle By Name(cluster=w313, "Timestamp"=w311) -> (w312:T1)
        n146 = case shown="False" w316 {
          tunnel: w315 -> [w324 _]
          tunnel: [w326 w328] -> w314
          tunnel: w312 -> [w327 w329]
          frame False {
            n147 = xnode ("FIFO Method Node")("Element"=w324, "Timeout"=0) -> ()  [unwired: 1 in, 2 out]
            n148 = Equal?(x=u8 127, y=w324) -> (x = y?=w322:bool)
            n149 = Select(t=VFDSampleSensorLoopStates."ReadFunction" ("InclinometerState"), s=w322, f=VFDSampleSensorLoopStates."ResponseAddressError" ("InclinometerState")) -> (s? t:f=w319:T2)
            n150 = Bundle By Name(cluster=w327, "State"=w319, "Timeout"=0) -> (w326:T1)
          }
          frame True {
            n151 = call "VFDCheckForTimeout.vi"("VFDSampleSensorLoopData in"=w329) -> ("VFDSampleSensorLoopData out"=w328:T1)  [unwired: 10 in]
          }
        }
      }
      frame "ReadFunction" {
        n152 = xnode ("FIFO Method Node")("Timeout"=0) -> ("Element"=w332:u8, "Timed Out?"=w333:bool)  [unwired: 1 in, 1 out]
        n153 = case shown="False" w333 {
          tunnel: w332 -> [w340 _]
          tunnel: [w347 w349] -> w331
          tunnel: w330 -> [w348 w350]
          frame False {
            n154 = xnode ("FIFO Method Node")("Element"=w340, "Timeout"=0) -> ()  [unwired: 1 in, 2 out]
            n155 = Equal?(x=u8 131, y=w340) -> (x = y?=w339:bool)
            n156 = Equal?(x=u8 3, y=w340) -> (x = y?=w344:bool)
            n157 = Select(t=VFDSampleSensorLoopStates."ReadExceptionCode" ("InclinometerState"), s=w339, f=VFDSampleSensorLoopStates."ResponseFunctionCodeError" ("InclinometerState")) -> (s? t:f=w342:T2)
            n158 = Select(t=VFDSampleSensorLoopStates."ReadByteCount" ("InclinometerState"), s=w344, f=w342) -> (s? t:f=w336:T2)
            n159 = Bundle By Name(cluster=w348, "State"=w336, "Timeout"=0) -> (w347:T1)
          }
          frame True {
            n160 = call "VFDCheckForTimeout.vi"("VFDSampleSensorLoopData in"=w350) -> ("VFDSampleSensorLoopData out"=w349:T1)  [unwired: 10 in]
          }
        }
      }
      frame "ReadByteCount" {
        n161 = xnode ("FIFO Method Node")("Timeout"=0) -> ("Element"=w353:u8, "Timed Out?"=w354:bool)  [unwired: 1 in, 1 out]
        n162 = case shown="False" w354 {
          tunnel: w353 -> [w362 _]
          tunnel: [w364 w366] -> w352
          tunnel: w351 -> [w365 w367]
          frame False {
            n163 = xnode ("FIFO Method Node")("Element"=w362, "Timeout"=0) -> ()  [unwired: 1 in, 2 out]
            n164 = Equal?(x=u8 14, y=w362) -> (x = y?=w360:bool)
            n165 = Select(t=VFDSampleSensorLoopStates."StartVelocityBits" ("InclinometerState"), s=w360, f=VFDSampleSensorLoopStates."ResponseByteCountError" ("InclinometerState")) -> (s? t:f=w357:T2)
            n166 = Bundle By Name(cluster=w365, "State"=w357, "Timeout"=0) -> (w364:T1)
          }
          frame True {
            n167 = call "VFDCheckForTimeout.vi"("VFDSampleSensorLoopData in"=w367) -> ("VFDSampleSensorLoopData out"=w366:T1)  [unwired: 10 in]
          }
        }
      }
      frame "StartVelocityBits" {
        n168 = Bundle By Name(cluster=w372, "State"=VFDSampleSensorLoopStates."ReadDataByte1", "StateAfterRead"=VFDSampleSensorLoopStates."EndVelocityBits", "U16"=u16 0 ("U32")) -> (w371:T1)
      }
      frame "EndVelocityBits" {
        n169 = Bundle By Name(cluster=w376, "State"=VFDSampleSensorLoopStates."StartDriveErrorBits", "Sample.VelocityBits"=w373) -> (w375:T1)
      }
      frame "StartDriveErrorBits" {
        n170 = Bundle By Name(cluster=w381, "State"=VFDSampleSensorLoopStates."ReadDataByte1", "StateAfterRead"=VFDSampleSensorLoopStates."EndDriveErrorBits", "U16"=u16 0 ("U32")) -> (w380:T1)
      }
      frame "EndDriveErrorBits" {
        n171 = Bundle By Name(cluster=w385, "State"=VFDSampleSensorLoopStates."StartFrequencyCommand", "Sample.DriveErrorBits"=w382) -> (w384:T1)
      }
      frame "StartFrequencyCommand" {
        n172 = Bundle By Name(cluster=w390, "State"=VFDSampleSensorLoopStates."ReadDataByte1", "StateAfterRead"=VFDSampleSensorLoopStates."EndFrequencyCommand", "U16"=u16 0 ("U32")) -> (w389:T1)
      }
      frame "EndFrequencyCommand" {
        n173 = Bundle By Name(cluster=w394, "State"=VFDSampleSensorLoopStates."StartOutputFrequency", "Sample.FrequencyCommand"=w391) -> (w393:T1)
      }
      frame "StartOutputFrequency" {
        n174 = Bundle By Name(cluster=w399, "State"=VFDSampleSensorLoopStates."ReadDataByte1", "StateAfterRead"=VFDSampleSensorLoopStates."EndOutputFrequency", "U16"=u16 0 ("U32")) -> (w398:T1)
      }
      frame "EndOutputFrequency" {
        n175 = Bundle By Name(cluster=w403, "State"=VFDSampleSensorLoopStates."StartDriveErrorBits", "Sample.OutputFrequency"=w400) -> (w402:T1)
      }
      frame "StartOutputCurrent" {
        n176 = Bundle By Name(cluster=w408, "State"=VFDSampleSensorLoopStates."ReadDataByte1", "StateAfterRead"=VFDSampleSensorLoopStates."EndOutputCurrent", "U16"=u16 0 ("U32")) -> (w407:T1)
      }
      frame "EndOutputCurrent" {
        n177 = Bundle By Name(cluster=w412, "State"=VFDSampleSensorLoopStates."StartDCBusVoltage", "Sample.OutputCurrent"=w409) -> (w411:T1)
      }
      frame "StartDCBusVoltage" {
        n178 = Bundle By Name(cluster=w417, "State"=VFDSampleSensorLoopStates."ReadDataByte1", "StateAfterRead"=VFDSampleSensorLoopStates."EndDCBusVoltage", "U16"=u16 0 ("U32")) -> (w416:T1)
      }
      frame "EndDCBusVoltage" {
        n179 = Bundle By Name(cluster=w421, "State"=VFDSampleSensorLoopStates."StartOutputVoltage", "Sample.DCBusVoltage"=w418) -> (w420:T1)
      }
      frame "StartOutputVoltage" {
        n180 = Bundle By Name(cluster=w426, "State"=VFDSampleSensorLoopStates."ReadDataByte1", "StateAfterRead"=VFDSampleSensorLoopStates."EndOutputVoltage", "U16"=u16 0 ("U32")) -> (w425:T1)
      }
      frame "EndOutputVoltage" {
        n181 = Bundle By Name(cluster=w430, "State"=VFDSampleSensorLoopStates."ReadCRCByte0", "Sample.OutputVoltage"=w427) -> (w429:T1)
      }
      frame "ReadDataByte1" {
        n182 = xnode ("FIFO Method Node")("Timeout"=0) -> ("Element"=w434:u8, "Timed Out?"=w435:bool)  [unwired: 1 in, 1 out]
        n183 = case shown="False" w435 {
          tunnel: w434 -> [w440 _]
          tunnel: [w448 w450] -> w433
          tunnel: w432 -> [w449 w451]
          tunnel: w431 -> [w444 _]
          frame False {
            n184 = To Unsigned Word Integer(number=w440) -> (unsigned 16bit integer=w439:u16)
            n185 = xnode ("FIFO Method Node")("Element"=w440, "Timeout"=0) -> ()  [unwired: 1 in, 2 out]
            n186 = Logical Shift(y=i16 8, x=w439) -> (x << y=w442:u16)
            n187 = And(x=u16 255, y=w444) -> (x .and. y?=w441:u16)
            n188 = Or(x=w441, y=w442) -> (x .or. y?=w438:u16)
            n189 = Bundle By Name(cluster=w449, "State"=VFDSampleSensorLoopStates."ReadDataByte0" ("InclinometerState"), "U16"=w438, "Timeout"=0) -> (w448:T1)
          }
          frame True {
            n190 = call "VFDCheckForTimeout.vi"("VFDSampleSensorLoopData in"=w451) -> ("VFDSampleSensorLoopData out"=w450:T1)  [unwired: 10 in]
          }
        }
      }
      frame "ReadDataByte0" {
        n191 = xnode ("FIFO Method Node")("Timeout"=0) -> ("Element"=w457:u8, "Timed Out?"=w453:bool)  [unwired: 1 in, 1 out]
        n192 = case shown="False" w453 {
          tunnel: w457 -> [w460 _]
          tunnel: [w470 w471] -> w456
          tunnel: w455 -> [w459 w472]
          tunnel: w454 -> [w468 _]
          frame False {
            n193 = To Unsigned Word Integer(number=w460) -> (unsigned 16bit integer=w464:u16)
            n194 = xnode ("FIFO Method Node")("Element"=w460, "Timeout"=0) -> ()  [unwired: 1 in, 2 out]
            n195 = Logical Shift(y=i16 0, x=w464) -> (x << y=w466:u16)
            n196 = And(x=u16 65280, y=w468) -> (x .and. y?=w465:u16)
            n197 = Or(x=w465, y=w466) -> (x .or. y?=w463:u16)
            n198 = Unbundle By Name(w459) -> ("StateAfterRead"=w458:T2)
            n199 = Bundle By Name(cluster=w459, "State"=w458, "U16"=w463, "Timeout"=0) -> (w470:T1)
          }
          frame True {
            n200 = call "VFDCheckForTimeout.vi"("VFDSampleSensorLoopData in"=w472) -> ("VFDSampleSensorLoopData out"=w471:T1)  [unwired: 10 in]
          }
        }
      }
      frame "Reserved1" {
        n201 = Bundle By Name(cluster=w474, "State"=VFDSampleSensorLoopStates."Reserved2" ("InclinometerState")) -> (w475:T1)
      }
      frame "Reserved2" {
        n202 = Bundle By Name(cluster=w477, "State"=VFDSampleSensorLoopStates."ReadCRCByte0") -> (w478:T1)
      }
      frame "ReadCRCByte0" {
        n203 = xnode ("FIFO Method Node")("Timeout"=0) -> ("Element"=w484:u8, "Timed Out?"=w479:bool)  [unwired: 1 in, 1 out]
        n204 = case shown="False" w479 {
          tunnel: w484 -> [w485 _]
          tunnel: [w495 w497] -> w483
          tunnel: w482 -> [w496 w498]
          tunnel: w481 -> [w487 _]
          frame False {
            n205 = To Unsigned Word Integer(number=w485) -> (unsigned 16bit integer=w489:u16)
            n206 = Logical Shift(y=i16 0, x=w489) -> (x << y=w491:u16)
            n207 = And(x=u16 65280, y=w487) -> (x .and. y?=w490:u16)
            n208 = Or(x=w490, y=w491) -> (x .or. y?=w488:u16)
            n209 = Bundle By Name(cluster=w496, "State"=VFDSampleSensorLoopStates."ReadCRCByte1" ("InclinometerState"), "CRC"=w488, "Timeout"=0) -> (w495:T1)
          }
          frame True {
            n210 = call "VFDCheckForTimeout.vi"("VFDSampleSensorLoopData in"=w498) -> ("VFDSampleSensorLoopData out"=w497:T1)  [unwired: 10 in]
          }
        }
      }
      frame "ReadCRCByte1" {
        n211 = xnode ("FIFO Method Node")("Timeout"=0) -> ("Element"=w504:u8, "Timed Out?"=w499:bool)  [unwired: 1 in, 1 out]
        n212 = case shown="False" w499 {
          tunnel: w504 -> [w505 _]
          tunnel: [w515 w517] -> w503
          tunnel: w502 -> [w516 w518]
          tunnel: w501 -> [w507 _]
          frame False {
            n213 = To Unsigned Word Integer(number=w505) -> (unsigned 16bit integer=w509:u16)
            n214 = Logical Shift(y=i16 8, x=w509) -> (x << y=w511:u16)
            n215 = And(x=u16 255, y=w507) -> (x .and. y?=w510:u16)
            n216 = Or(x=w510, y=w511) -> (x .or. y?=w508:u16)
            n217 = Bundle By Name(cluster=w516, "State"=VFDSampleSensorLoopStates."CalculateCRC" ("InclinometerState"), "CRC"=w508, "Timeout"=0) -> (w515:T1)
          }
          frame True {
            n218 = call "VFDCheckForTimeout.vi"("VFDSampleSensorLoopData in"=w518) -> ("VFDSampleSensorLoopData out"=w517:T1)  [unwired: 10 in]
          }
        }
      }
      frame "CalculateCRC" {
        n219 = xnode ("FIFO Method Node")("Element"=TRUE, "Timeout"=0) -> ()  [unwired: 1 in, 2 out]
        n220 = Bundle By Name(cluster=w522, "State"=VFDSampleSensorLoopStates."ValidateCRC" ("InclinometerState")) -> (w523:T1)
      }
      frame "ValidateCRC" {
        n221 = xnode ("FIFO Method Node")("Timeout"=0) -> ("Element"=w529:u16, "Timed Out?"=w524:bool)  [unwired: 1 in, 1 out]
        n222 = case shown="False" w524 {
          tunnel: w529 -> [w530 _]
          tunnel: [w538 w540] -> w528
          tunnel: w527 -> [w539 w540]
          tunnel: w526 -> [w533 _]
          frame False {
            n223 = xnode ("Register Read")() -> ("Data"=w532:u64)  [unwired: 1 in, 1 out]
            n224 = Equal?(x=w533, y=w530) -> (x = y?=w537:bool)
            n225 = Select(t=VFDSampleSensorLoopStates."PrepareSample" ("InclinometerState"), s=w537, f=VFDSampleSensorLoopStates."ResponseCRCError" ("InclinometerState")) -> (s? t:f=w534:T2)
            n226 = Increment(x=w532) -> (x+1=w531:u64)
            n227 = xnode ("Register Write")("Data"=w531) -> ()  [unwired: 1 in, 1 out]
            n228 = Bundle By Name(cluster=w539, "State"=w534) -> (w538:T1)
          }
          frame True {
          }
        }
      }
      frame "PrepareSample" {
        n229 = xnode ("Register Read")() -> ("Data"=w544:u64)  [unwired: 1 in, 1 out]
        n230 = xnode ("Register Read")() -> ("Data"=w543:u64)  [unwired: 1 in, 1 out]
        n231 = xnode ("Register Read")() -> ("Data"=w542:u64)  [unwired: 1 in, 1 out]
        n232 = xnode ("Register Read")() -> ("Data"=w541:u64)  [unwired: 1 in, 1 out]
        n233 = Bundle By Name(cluster=w547, "State"=VFDSampleSensorLoopStates."MoveSample", "Sample.Timestamp"=w546, "Sample.TxBytes"=w544, "Sample.RxBytes"=w543, "Sample.TxFrames"=w542, "Sample.RxFrames"=w541) -> (w548:T1)
      }
      frame "MoveSample" {
        n234 = xnode ("FIFO Method Node")("Element"=w549, "Timeout"=0) -> ()  [unwired: 1 in, 2 out]
        n235 = Bundle By Name(cluster=w552, "State"=VFDSampleSensorLoopStates."WaitForTrigger") -> (w553:T1)
      }
      frame "ReadExceptionCode" {
        n236 = xnode ("FIFO Method Node")("Timeout"=0) -> ("Element"=w558:u8, "Timed Out?"=w554:bool)  [unwired: 1 in, 1 out]
        n237 = case shown="False" w554 {
          tunnel: w558 -> [w559 _]
          tunnel: [w570 w572] -> w557
          tunnel: w556 -> [w571 w573]
          frame False {
            n238 = xnode ("FIFO Method Node")("Element"=w559, "Timeout"=0) -> ()  [unwired: 1 in, 2 out]
            n239 = Equal?(x=u8 1, y=w559) -> (x = y?=w563:bool)
            n240 = Equal?(x=u8 2, y=w559) -> (x = y?=w562:bool)
            n241 = Or(x=w563, y=w562) -> (x .or. y?=w561:bool)
            n242 = Select(t=VFDSampleSensorLoopStates."ReadExceptionCRCByte0" ("InclinometerState"), s=w561, f=VFDSampleSensorLoopStates."ResponseUnknownError" ("InclinometerState")) -> (s? t:f=w566:T2)
            n243 = Bundle By Name(cluster=w571, "State"=w566, "Timeout"=0, "Exception"=w559) -> (w570:T1)
          }
          frame True {
            n244 = call "VFDCheckForTimeout.vi"("VFDSampleSensorLoopData in"=w573) -> ("VFDSampleSensorLoopData out"=w572:T1)  [unwired: 10 in]
          }
        }
      }
      frame "ReadExceptionCRCByte0" {
        n245 = xnode ("FIFO Method Node")("Timeout"=0) -> ("Element"=w579:u8, "Timed Out?"=w574:bool)  [unwired: 1 in, 1 out]
        n246 = case shown="False" w574 {
          tunnel: w579 -> [w580 _]
          tunnel: [w590 w592] -> w578
          tunnel: w577 -> [w591 w593]
          tunnel: w576 -> [w582 _]
          frame False {
            n247 = To Unsigned Word Integer(number=w580) -> (unsigned 16bit integer=w584:u16)
            n248 = Logical Shift(y=i16 0, x=w584) -> (x << y=w586:u16)
            n249 = And(x=u16 65280, y=w582) -> (x .and. y?=w585:u16)
            n250 = Or(x=w585, y=w586) -> (x .or. y?=w583:u16)
            n251 = Bundle By Name(cluster=w591, "State"=VFDSampleSensorLoopStates."ReadExceptionCRCByte1" ("InclinometerState"), "CRC"=w583, "Timeout"=0) -> (w590:T1)
          }
          frame True {
            n252 = call "VFDCheckForTimeout.vi"("VFDSampleSensorLoopData in"=w593) -> ("VFDSampleSensorLoopData out"=w592:T1)  [unwired: 10 in]
          }
        }
      }
      frame "ReadExceptionCRCByte1" {
        n253 = xnode ("FIFO Method Node")("Timeout"=0) -> ("Element"=w599:u8, "Timed Out?"=w594:bool)  [unwired: 1 in, 1 out]
        n254 = case shown="False" w594 {
          tunnel: w599 -> [w600 _]
          tunnel: [w610 w612] -> w598
          tunnel: w597 -> [w611 w613]
          tunnel: w596 -> [w602 _]
          frame False {
            n255 = To Unsigned Word Integer(number=w600) -> (unsigned 16bit integer=w604:u16)
            n256 = Logical Shift(y=i16 8, x=w604) -> (x << y=w606:u16)
            n257 = And(x=u16 255, y=w602) -> (x .and. y?=w605:u16)
            n258 = Or(x=w605, y=w606) -> (x .or. y?=w603:u16)
            n259 = Bundle By Name(cluster=w611, "State"=VFDSampleSensorLoopStates."CalculateExceptionCRC" ("InclinometerState"), "CRC"=w603, "Timeout"=0) -> (w610:T1)
          }
          frame True {
            n260 = call "VFDCheckForTimeout.vi"("VFDSampleSensorLoopData in"=w613) -> ("VFDSampleSensorLoopData out"=w612:T1)  [unwired: 10 in]
          }
        }
      }
      frame "CalculateExceptionCRC" {
        n261 = xnode ("FIFO Method Node")("Element"=TRUE, "Timeout"=0) -> ()  [unwired: 1 in, 2 out]
        n262 = Bundle By Name(cluster=w617, "State"=VFDSampleSensorLoopStates."ValidateExceptionCRC" ("InclinometerState")) -> (w618:T1)
      }
      frame "ValidateExceptionCRC" {
        n263 = xnode ("FIFO Method Node")("Timeout"=0) -> ("Element"=w624:u16, "Timed Out?"=w619:bool)  [unwired: 1 in, 1 out]
        n264 = case shown="False" w619 {
          tunnel: w624 -> [w625 _]
          tunnel: [w633 w635] -> w623
          tunnel: w622 -> [w634 w635]
          tunnel: w621 -> [w628 _]
          frame False {
            n265 = xnode ("Register Read")() -> ("Data"=w627:u64)  [unwired: 1 in, 1 out]
            n266 = Equal?(x=w628, y=w625) -> (x = y?=w632:bool)
            n267 = Select(t=VFDSampleSensorLoopStates."ParseExceptionCode" ("InclinometerState"), s=w632, f=VFDSampleSensorLoopStates."ResponseCRCError" ("InclinometerState")) -> (s? t:f=w629:T2)
            n268 = Increment(x=w627) -> (x+1=w626:u64)
            n269 = xnode ("Register Write")("Data"=w626) -> ()  [unwired: 1 in, 1 out]
            n270 = Bundle By Name(cluster=w634, "State"=w629) -> (w633:T1)
          }
          frame True {
          }
        }
      }
      frame "ParseExceptionCode" {
        n271 = Equal?(x=w637, y=u8 1) -> (x = y?=w641:bool)
        n272 = Select(t=VFDSampleSensorLoopStates."SensorReportsIllegalFunction" ("InclinometerState"), s=w641, f=VFDSampleSensorLoopStates."SensorReportsIllegalDataAddress" ("InclinometerState")) -> (s? t:f=w638:T2)
        n273 = Bundle By Name(cluster=w642, "State"=w638) -> (w643:T1)
      }
      frame "ResponseAddressError" {
        n274 = Bundle By Name(cluster=w646, "State"=VFDSampleSensorLoopStates."PrepareErrorCode" ("InclinometerState"), "ErrorSample.ErrorCode"=VFDErrorCodes."ResponseAddressError" ("InclinometerErrorCodes")) -> (w647:T1)
      }
      frame "ResponseFunctionCodeError" {
        n275 = Bundle By Name(cluster=w650, "State"=VFDSampleSensorLoopStates."PrepareErrorCode" ("InclinometerState"), "ErrorSample.ErrorCode"=VFDErrorCodes."ResponseFunctionCodeError" ("InclinometerErrorCodes")) -> (w651:T1)
      }
      frame "ResponseByteCountError" {
        n276 = Bundle By Name(cluster=w654, "State"=VFDSampleSensorLoopStates."PrepareErrorCode" ("InclinometerState"), "ErrorSample.ErrorCode"=VFDErrorCodes."ResponseByteCountError" ("InclinometerErrorCodes")) -> (w655:T1)
      }
      frame "ResponseCRCError" {
        n277 = Bundle By Name(cluster=w658, "State"=VFDSampleSensorLoopStates."PrepareErrorCode" ("InclinometerState"), "ErrorSample.ErrorCode"=VFDErrorCodes."ResponseCRCError" ("InclinometerErrorCodes")) -> (w659:T1)
      }
      frame "ResponseUnknownError" {
        n278 = Bundle By Name(cluster=w662, "State"=VFDSampleSensorLoopStates."PrepareErrorCode" ("InclinometerState"), "ErrorSample.ErrorCode"=VFDErrorCodes."ResponseUnknownError" ("InclinometerErrorCodes")) -> (w663:T1)
      }
      frame "ResponseTimeoutError" {
        n279 = Bundle By Name(cluster=w666, "State"=VFDSampleSensorLoopStates."PrepareErrorCode" ("InclinometerState"), "ErrorSample.ErrorCode"=VFDErrorCodes."ResponseTimeoutError" ("InclinometerErrorCodes")) -> (w667:T1)
      }
      frame "SensorReportsIllegalFunction" {
        n280 = Bundle By Name(cluster=w670, "State"=VFDSampleSensorLoopStates."PrepareErrorCode" ("InclinometerState"), "ErrorSample.ErrorCode"=VFDErrorCodes."SensorReportsIllegalFunction" ("InclinometerErrorCodes")) -> (w671:T1)
      }
      frame "SensorReportsIllegalDataAddress" {
        n281 = Bundle By Name(cluster=w674, "State"=VFDSampleSensorLoopStates."PrepareErrorCode" ("InclinometerState"), "ErrorSample.ErrorCode"=VFDErrorCodes."SensorReportsIllegalDataAddress" ("InclinometerErrorCodes")) -> (w675:T1)
      }
      frame "PrepareErrorCode" {
        n282 = xnode ("Register Read")() -> ("Data"=w679:u64)  [unwired: 1 in, 1 out]
        n283 = xnode ("Register Read")() -> ("Data"=w678:u64)  [unwired: 1 in, 1 out]
        n284 = xnode ("Register Read")() -> ("Data"=w677:u64)  [unwired: 1 in, 1 out]
        n285 = xnode ("Register Read")() -> ("Data"=w676:u64)  [unwired: 1 in, 1 out]
        n286 = Bundle By Name(cluster=w682, "State"=VFDSampleSensorLoopStates."MoveErrorCode", "ErrorSample.Timestamp"=w681, "ErrorSample.TxBytes"=w679, "ErrorSample.RxBytes"=w678, "ErrorSample.TxFrames"=w677, "ErrorSample.RxFrames"=w676) -> (w683:T1)
      }
      frame "MoveErrorCode" {
        n287 = xnode ("FIFO Method Node")("Element"=w685, "Timeout"=0) -> ()  [unwired: 1 in, 2 out]
        n288 = Bundle By Name(cluster=w687, "State"=VFDSampleSensorLoopStates."WaitForTrigger") -> (w688:T1)
      }
    }
  }
  n289 = node-c288(w2) -> ()
